vi "R and X plane.vi"(8 "inc":dbl=0.6 format="%#_13g", 9 "R0,X0":dbl=0.1 format="%#_13g", 11 "loops":i32=1) -> (1 "R":cluster{dbl[], dbl[]}[](graph), 2 "X":cluster{"x":dbl[], dbl[]}[](graph), 3 "loops":i32)   [LabVIEW 2014]
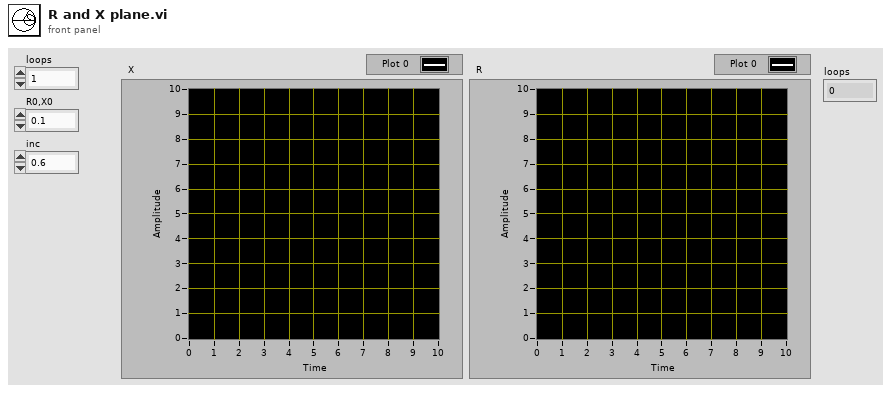
[diagram p1: front panel]
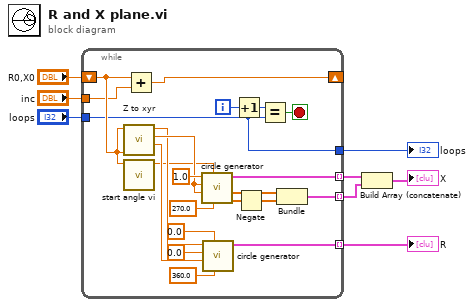
[diagram p0: block diagram]
diagram:
  n1 = while {
    tunnel: [w26] -> w7 mode=indexing
    tunnel: [w17] -> w4 mode=indexing
    tunnel: [w23] -> w8 mode=indexing
    shift-right: [w12] -> _
    shift-left: "R0,X0" -> [w11]
    tunnel: "inc" -> [w10]
    tunnel: "loops" -> [w9]
    tunnel: [w9] -> w1
    i -> [w30]
    stop <- w29 stop-if-true
    n2 = call "Z to xyr.vi"("Z"=w11, "R"=w11) -> ("r"=w15:dbl, "r/yc"=w16:dbl, "xc"=w14:dbl)  [unwired: 7 in]
    n3 = call "start angle vi.vi"("X"=w11) -> ("theta0"=w13:dbl)  [unwired: 10 in]
    n4 = Add(x=w11, y=w10) -> (x+y=w12:dbl)
    n5 = call "circle generator.vi"("end"=270.0 ("theta2/deg"), "start"=w13, "r"=w16, "yc"=w16, "xc"=1.0 ("yc")) -> ("y"=w22:dbl[], "x"=w21:dbl[], "graph"=w23:cluster{dbl[], dbl[]})  [unwired: 4 in]
    n6 = call "circle generator.vi"("end"=360.0 ("theta2/deg"), "start"=0.0, "r"=w15, "yc"=0.0 ("start"), "xc"=w14) -> ("graph"=w17:cluster{dbl[], dbl[]})  [unwired: 4 in, 2 out]
    n7 = Increment(x=w30) -> (x+1=w28:i32)
    n8 = Negate(x=w22) -> (-x=w27:dbl[])
    n9 = Equal?(x=w28, y=w9) -> (x = y?=w29:bool)
    n10 = Bundle("x"=w21, w27) -> (w26:cluster{"x":dbl[], dbl[]})  [unwired: 1 in]
  }
  "R" <- w4
  "loops" <- w1
  n11 = Build Array (concatenate)(w8, w7) -> (→"X":cluster{"x":dbl[], dbl[]}[])
